vi "13 Events.vi"() -> ()   [LabVIEW 2019]
uses:
  _Subs/OpenDiagram/Open_XControl.xctl
panel:
  in  "OpenDiag":refnum<vi>(xcontrol)
  out "job":string
  in  "Dial":dbl(knob) scale=0.0..10.0
  in  "Numeric":dbl
  in  "stop":bool
  # "12 Events\nEvents are a powerful way to build a UI - watch how the code executes.\n\nInstructions:\n1. Hit the Run arrow and see the the string change based on your button choice."
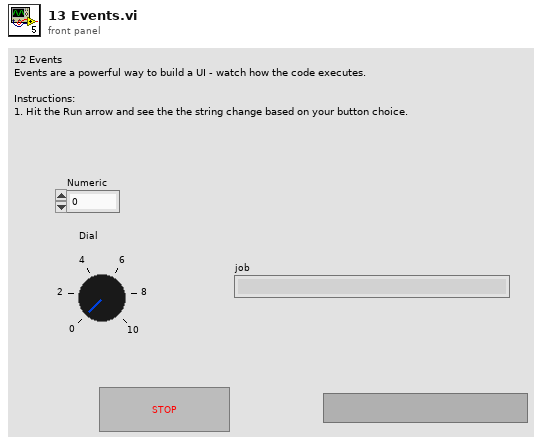
[diagram p1: front panel]
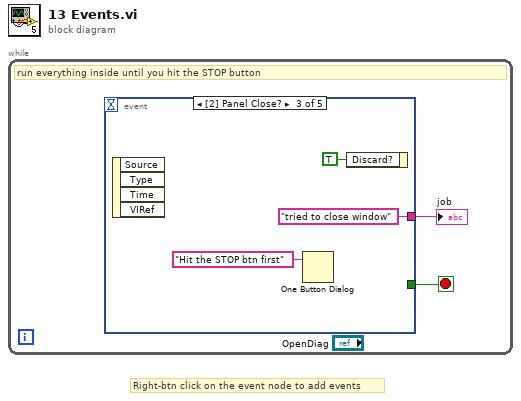
[diagram p0: block diagram]
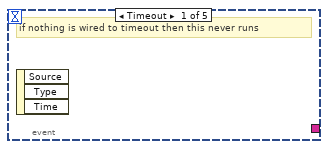
[diagram p2: hidden frame]
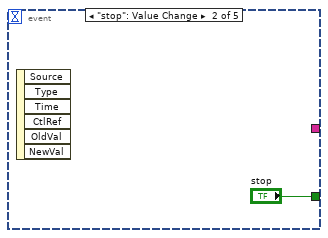
[diagram p3: hidden frame]
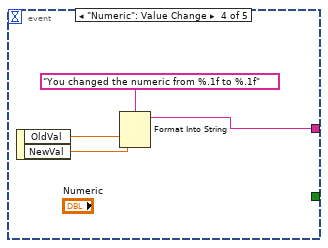
[diagram p4: hidden frame]
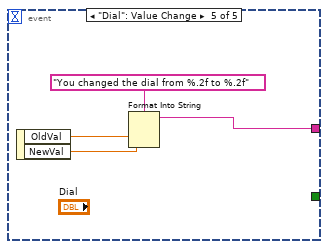
[diagram p5: hidden frame]
diagram:
  # "Right-btn click on the event node to add events"
  n1 = while {
    stop <- w2 stop-if-true
    # "run everything inside until you hit the STOP button"
    n2 = event shown="[2] Panel Close?" {
      selector: _ -> [_ _ _ _ _]
      dyn-events: _ -> [_ _ _ _ _]
      timeout: _ -> [_ _ _ _ _]
      tunnel: [_ "stop" _ _ _] -> w2
      tunnel: [_ _ "tried to close window" w7 w11] -> w1
      event Timeout {
        # "if nothing is wired to timeout then this never runs"
        n3 = event-data() -> ()  [unwired: 1 in, 3 out]
      }
      event "stop": Value Change {
        n4 = event-data() -> ()  [unwired: 1 in, 6 out]
      }
      event Panel Close? {
        n5 = event-data() -> ()  [unwired: 1 in, 4 out]
        n6 = One Button Dialog(message="Hit the STOP btn first") -> ()  [unwired: 1 in, 1 out]
        n7 = event-data("Discard?"=TRUE) -> ()  [unwired: 1 in, 1 out]
      }
      event "Numeric": Value Change {
        n8 = event-data() -> ("OldVal"=w9:dbl, "NewVal"=w8:dbl)  [unwired: 1 in]
        n9 = Format Into String(format string="You changed the numeric from %.1f to %.1f", w9, w8) -> (resulting string=w7:string)  [unwired: 2 in, 1 out]
      }
      event "Dial": Value Change {
        n10 = event-data() -> ("OldVal"=w13:dbl, "NewVal"=w12:dbl)  [unwired: 1 in]
        n11 = Format Into String(format string="You changed the dial from %.2f to %.2f", w13, w12) -> (resulting string=w11:string)  [unwired: 2 in, 1 out]
      }
    }
    "job" <- w1
  }
